vi "DeviceConnect.vi"(3 "VISA resource name 3":string, 4 "VISA resource name 2":string, 5 "VISA resource name":string) -> (0 "Multimeter":refnum<visa-resource-name>, 1 "Commutator":refnum<visa-resource-name>, 2 "Power Source":refnum<visa-resource-name>)   [LabVIEW 2021]
panel:
  out "error out":errorcluster
  in  "error in":errorcluster
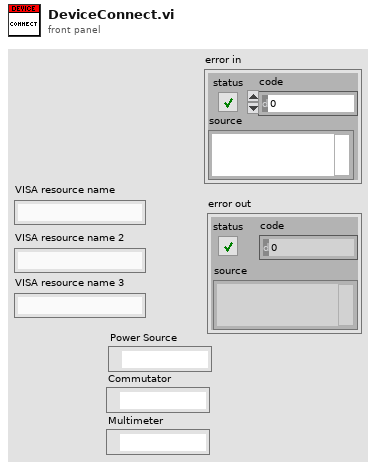
[diagram p1: front panel]
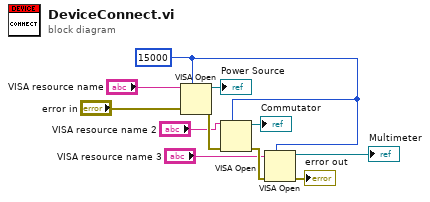
[diagram p0: block diagram]
diagram:
  w2 = u32 15000 ("VISA Open timeout (1000)")
  n1 = VISA Open(timeout (0)=w2, error in (no error)="error in", VISA resource name="VISA resource name") -> (VISA resource name=→"Power Source":refnum<visa-resource-name>, error out=w10:errorcluster)  [unwired: 2 in]
  n2 = VISA Open(timeout (0)=w2, error in (no error)=w10, VISA resource name="VISA resource name 2") -> (VISA resource name=→"Commutator":refnum<visa-resource-name>, error out=w9:errorcluster)  [unwired: 2 in]
  n3 = VISA Open(timeout (0)=w2, error in (no error)=w9, VISA resource name="VISA resource name 3") -> (VISA resource name=→"Multimeter":refnum<visa-resource-name>, error out=→"error out":errorcluster)  [unwired: 2 in]
